vi "PAQ-Defragment.vi"() -> ()   [LabVIEW 2020, in "Sgraph_lib_V1.lvlib"]
uses:
  Builds/Sgraph_lib_V1.lvlib
  Controls/BIN-PAQ-Defrag-Attributes.ctl
  DBAL/controls/BIN/BINdata.ctl
  DBAL/DBAL-BIN.lvclass
panel:
  in  "Save Defragmented Files":bool
  out "error out":errorcluster
  out "XY Graph":cluster{dbl[], "data":dbl[]}(graph)
  out "Segments":string
  out "File name":string
  out "Folder name":string
  out "Table type":string
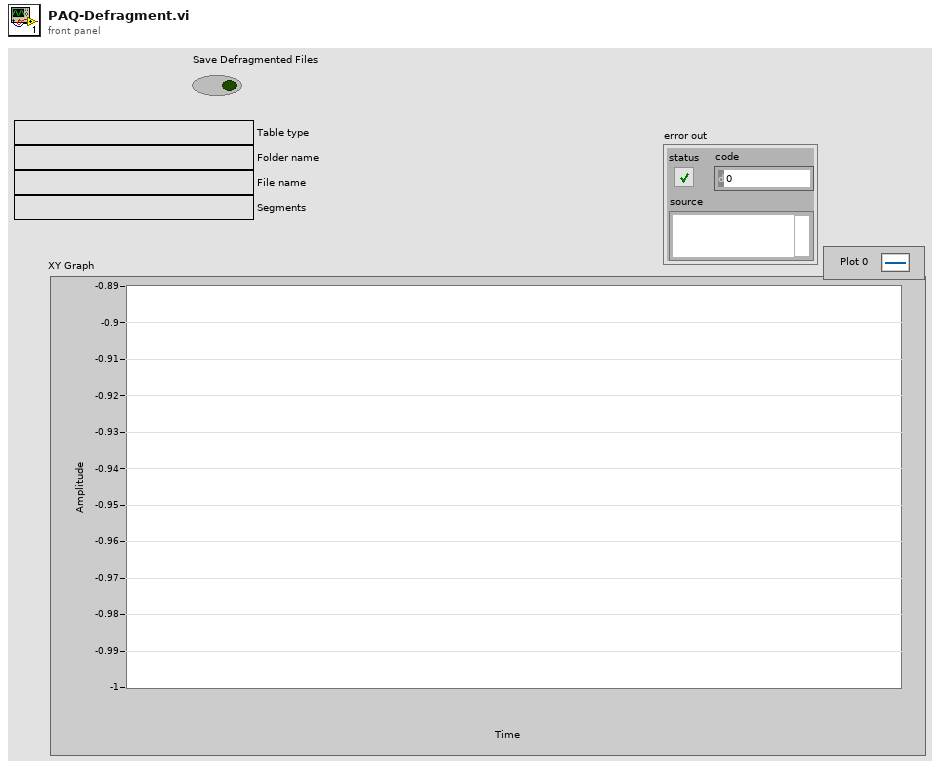
[diagram p1: front panel]
types:
  T1 = typedef "Sgraph_lib_V1.lvlib/BIN-PAQ-Defrag-Attributes.ctl" = cluster{"Database location":path, "Table Names":string[], "Ext":string, "WeekFolderNumbers":i32[], "FileDateNumbers":u64[], "WeekFolder":path, "HistFile":path, "BinHistData":T2, "Save Data":bool, "TAGs":string[], "Segments":i32}
  T2 = typedef "Sgraph_lib_V1.lvlib/DBAL-BIN.lvclass/BINdata.ctl" = cluster{"time":dbl[], "TagsData":cluster{"data":dbl[], "max":dbl[], "min":dbl[], "status":u32[]}[]}
  T3 = cluster{"data":dbl[], "max":dbl[], "min":dbl[], "status":u32[]}[]
  T4 = cluster{"data":dbl[], "max":dbl[], "min":dbl[], "status":u32[]}
  T5 = cluster{"TableName":string, "Data2save":cluster{"TAGs":string[], "time":dbl[], "TagsData":cluster{"data":dbl[], "max":dbl[], "min":dbl[], "status":u32[]}[]}}
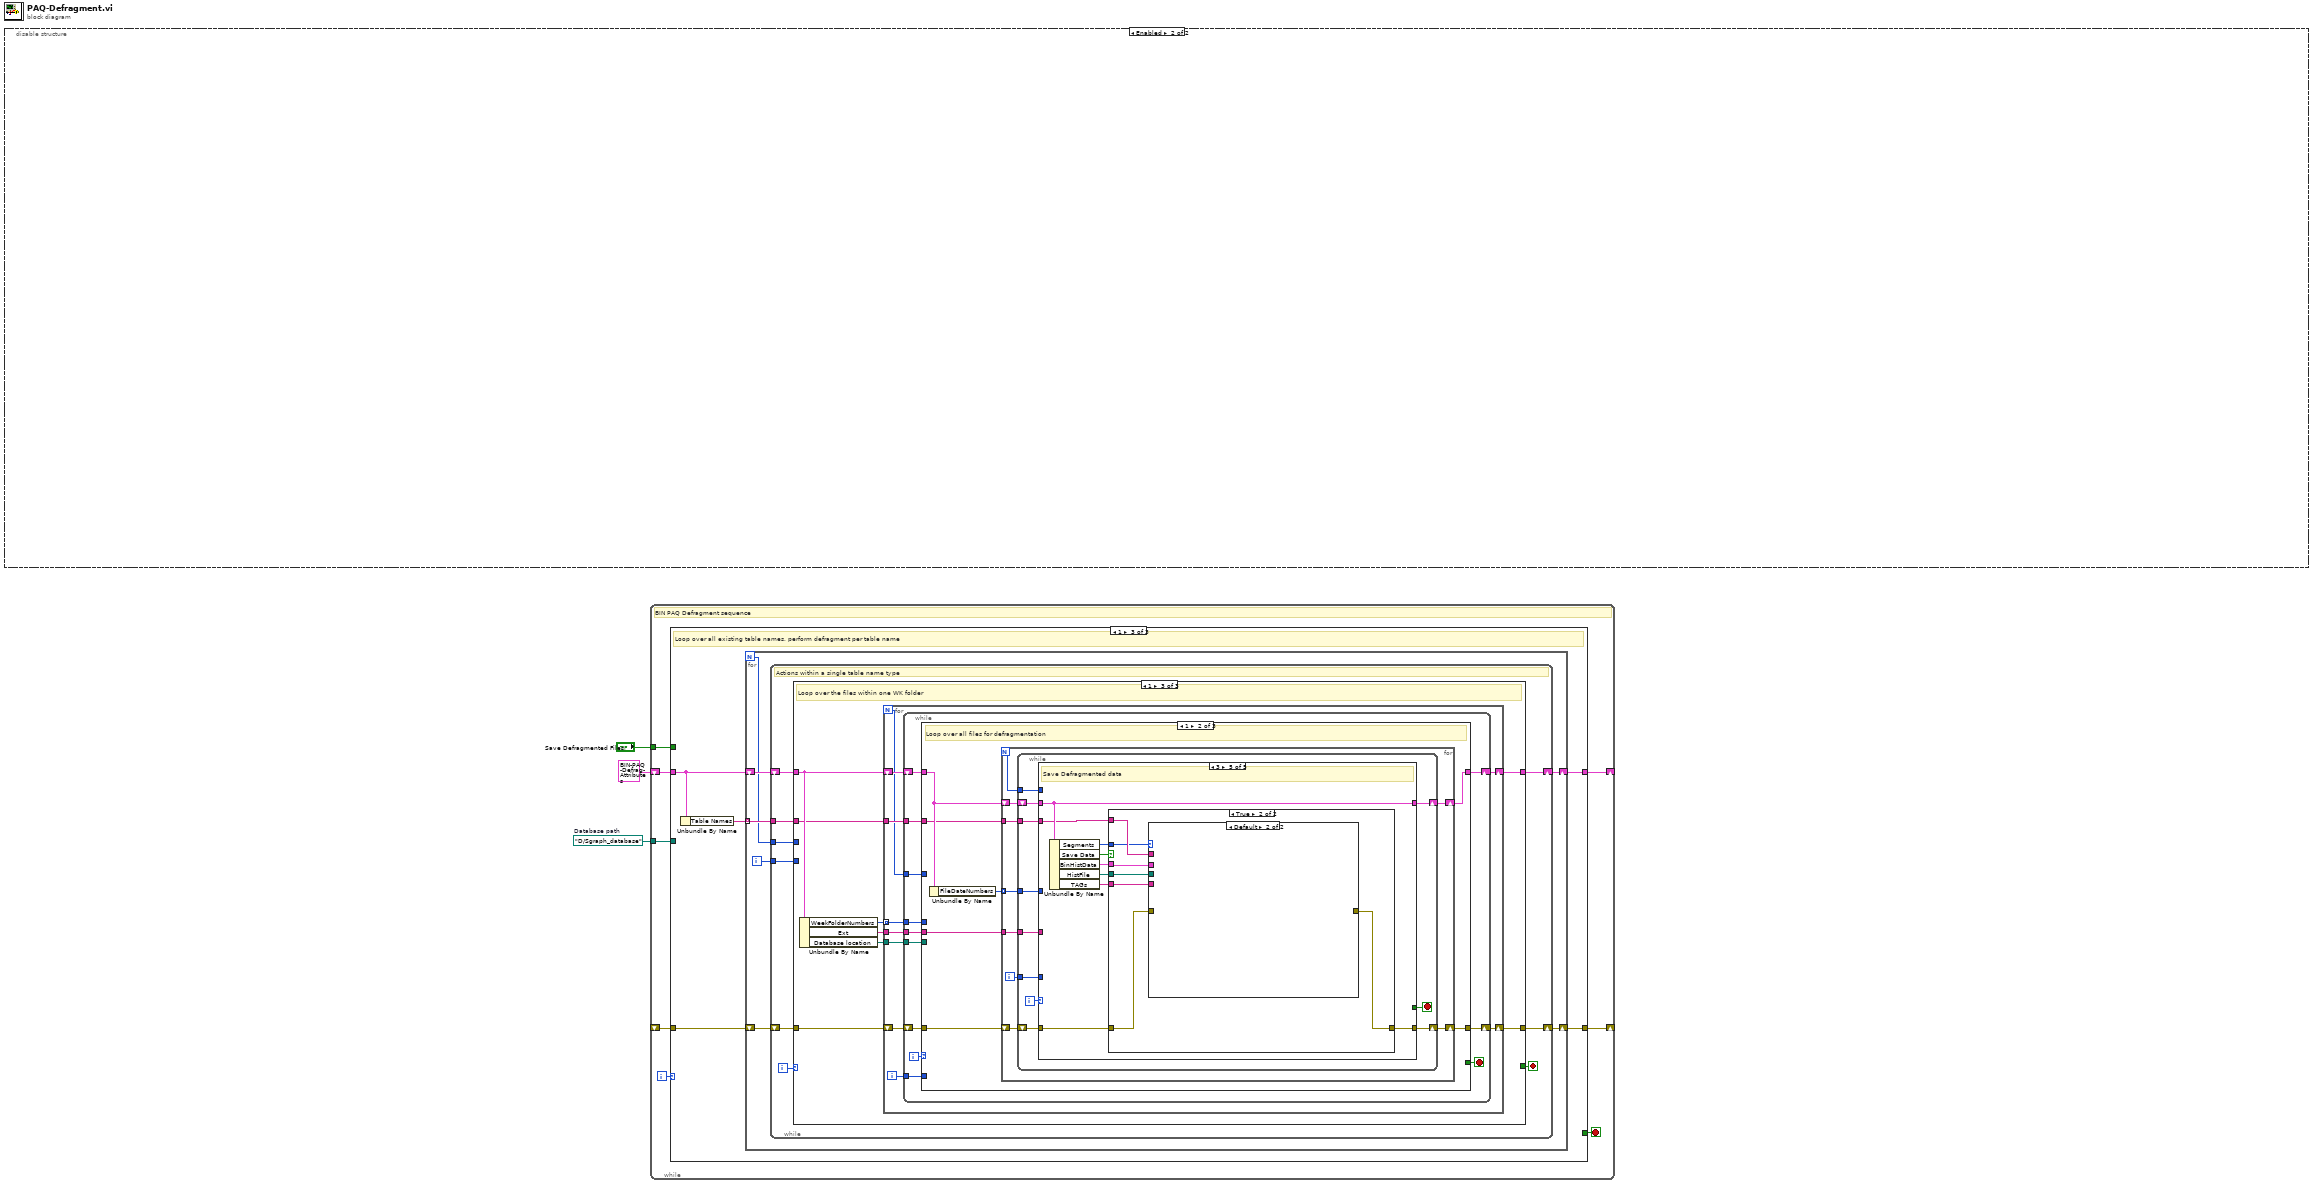
[diagram p0: block diagram]
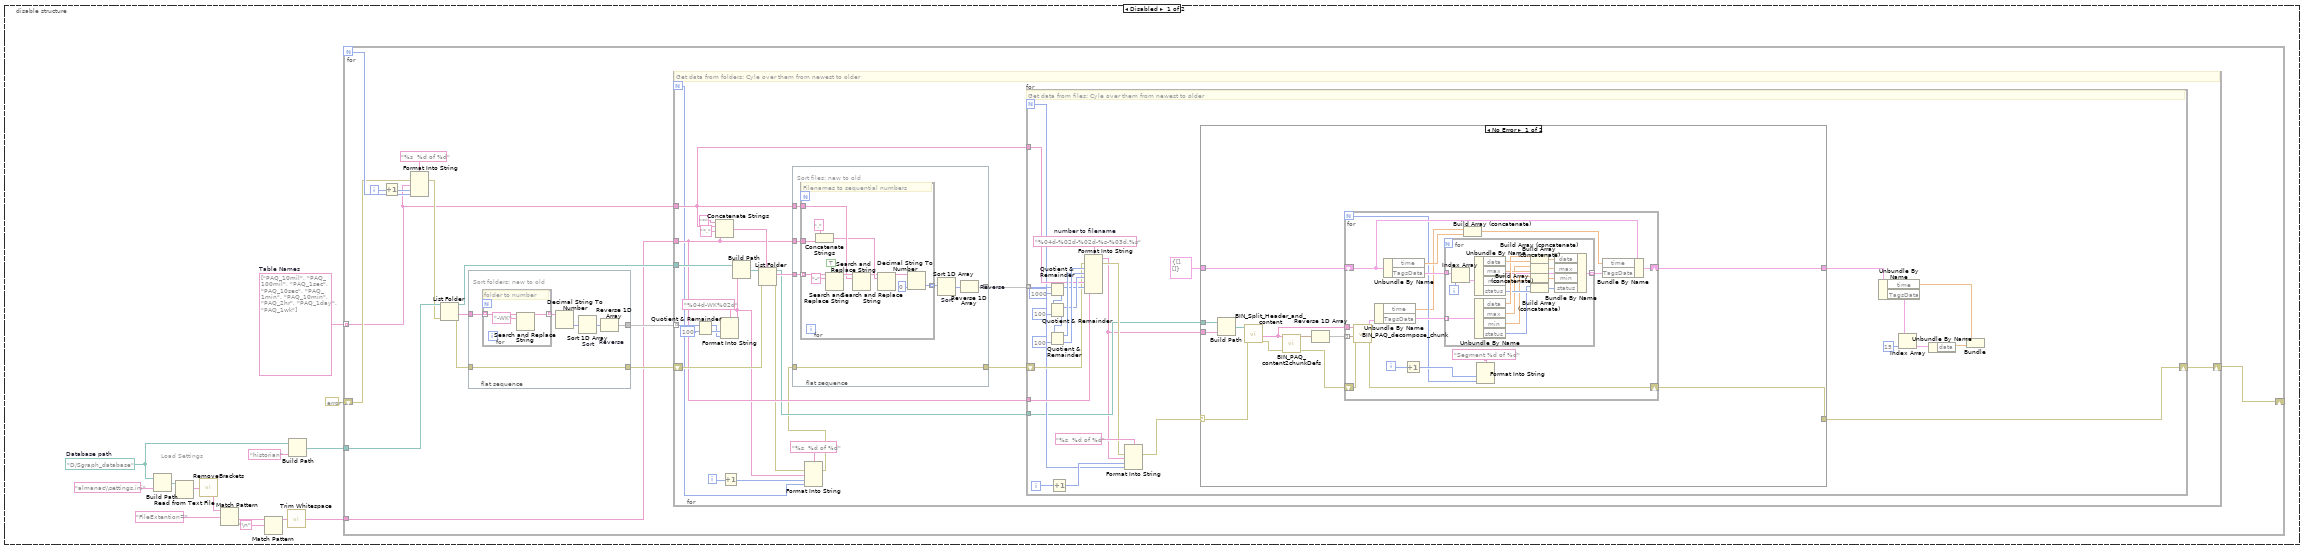
[diagram p2: hidden frame]
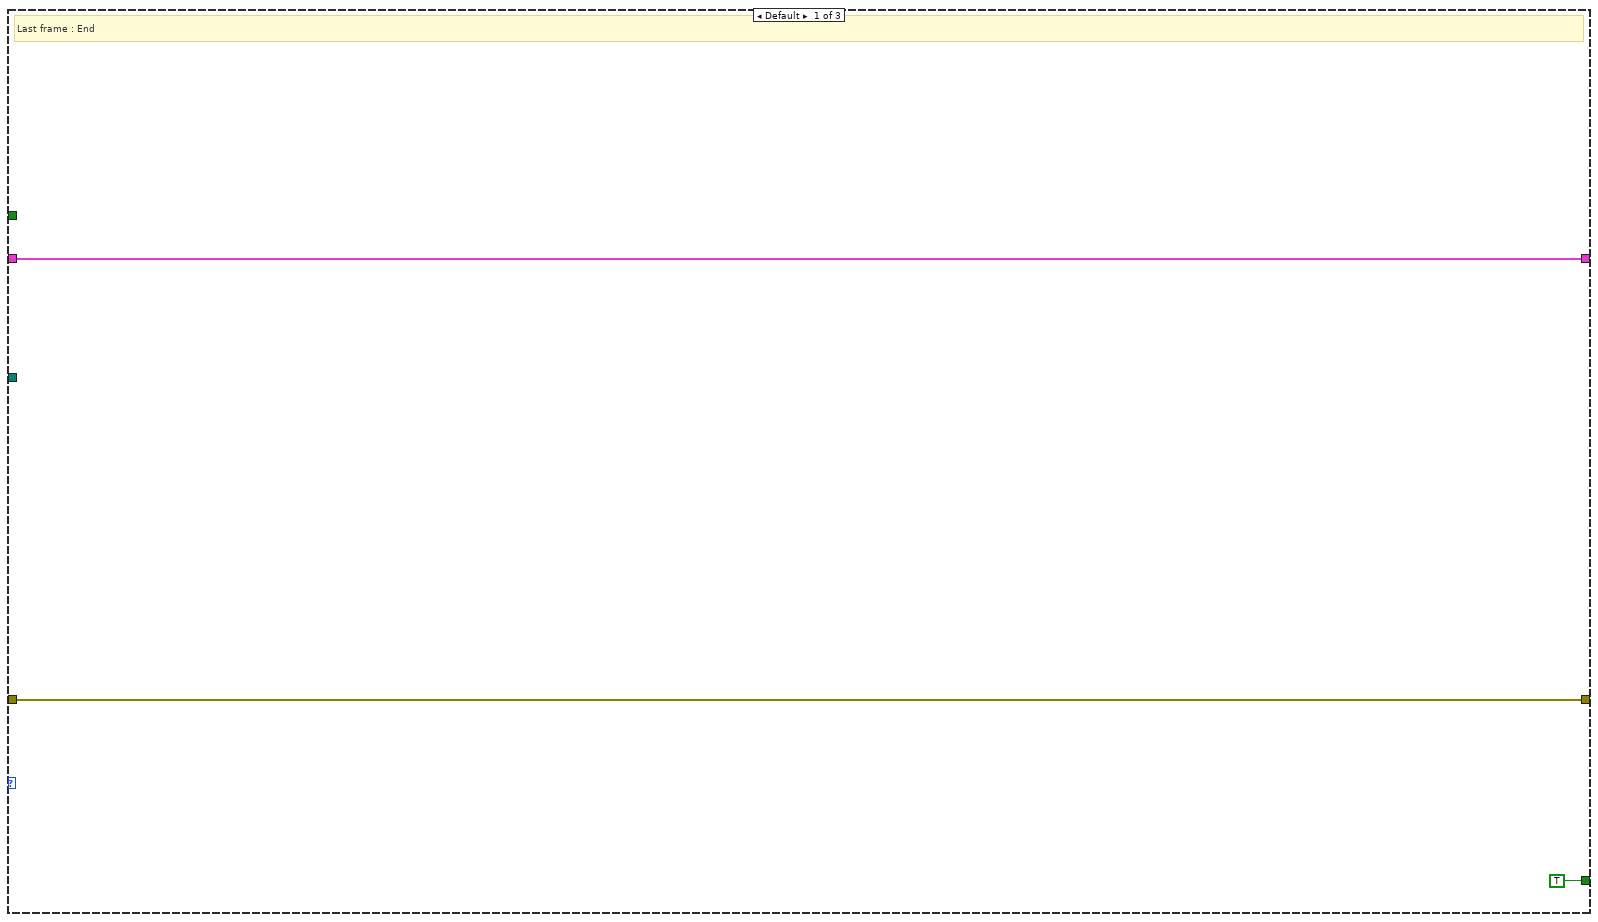
[diagram p4: hidden frame]
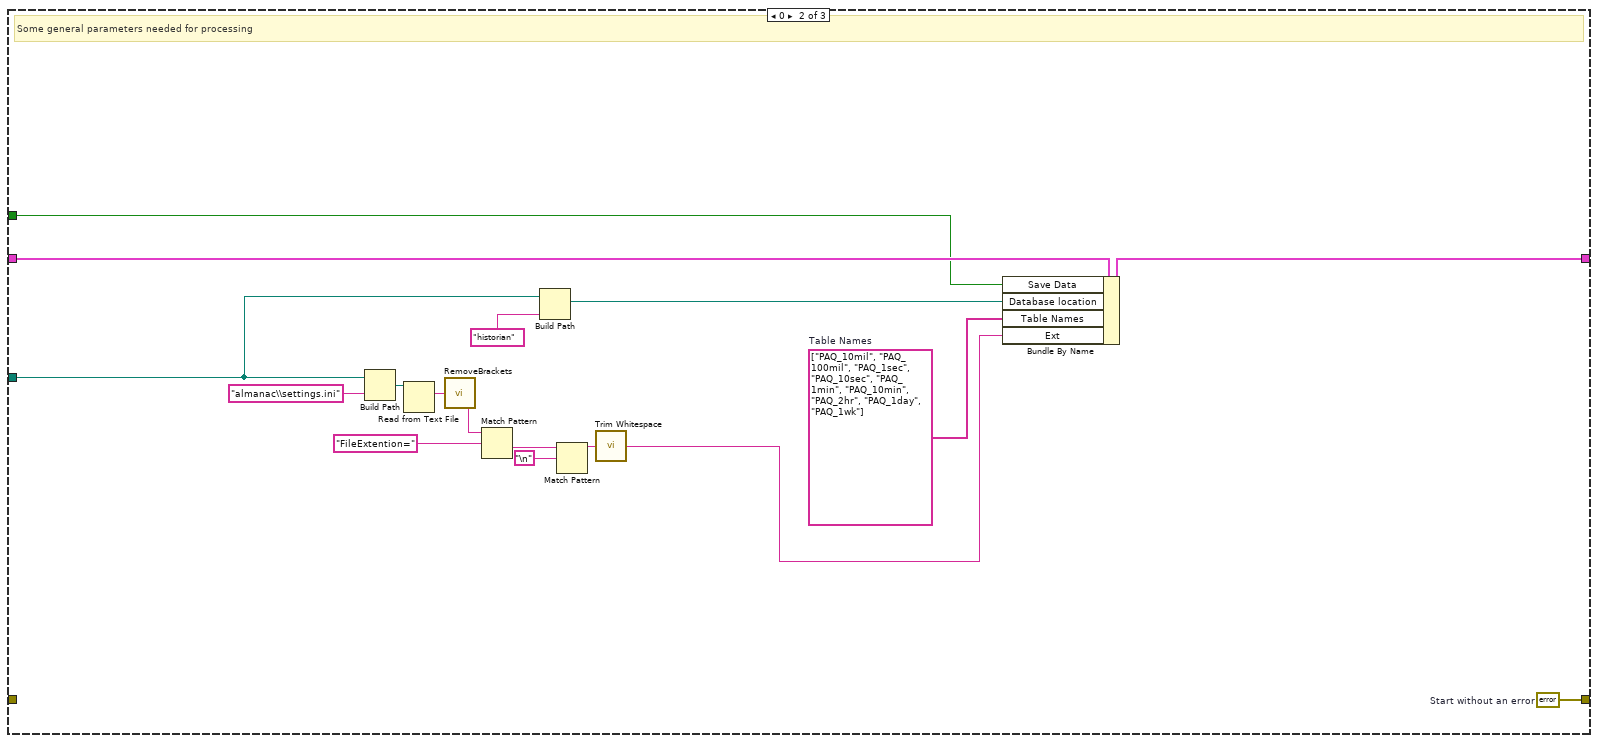
[diagram p5: hidden frame]
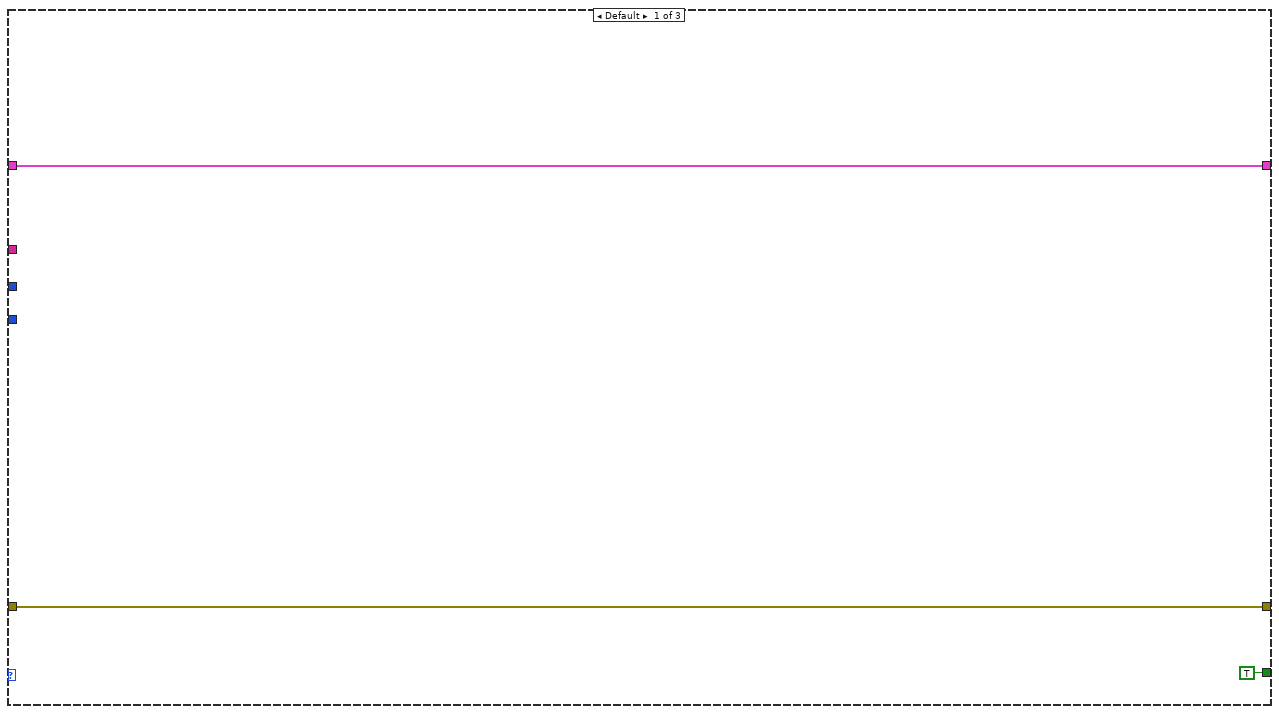
[diagram p6: hidden frame]
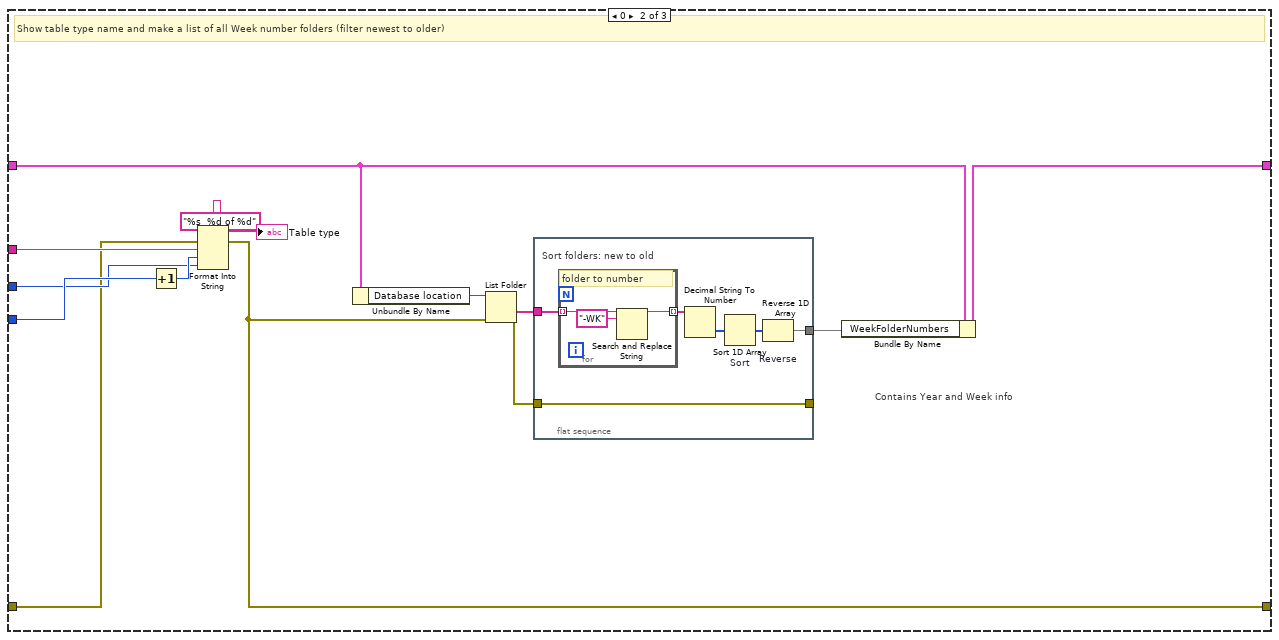
[diagram p7: hidden frame]
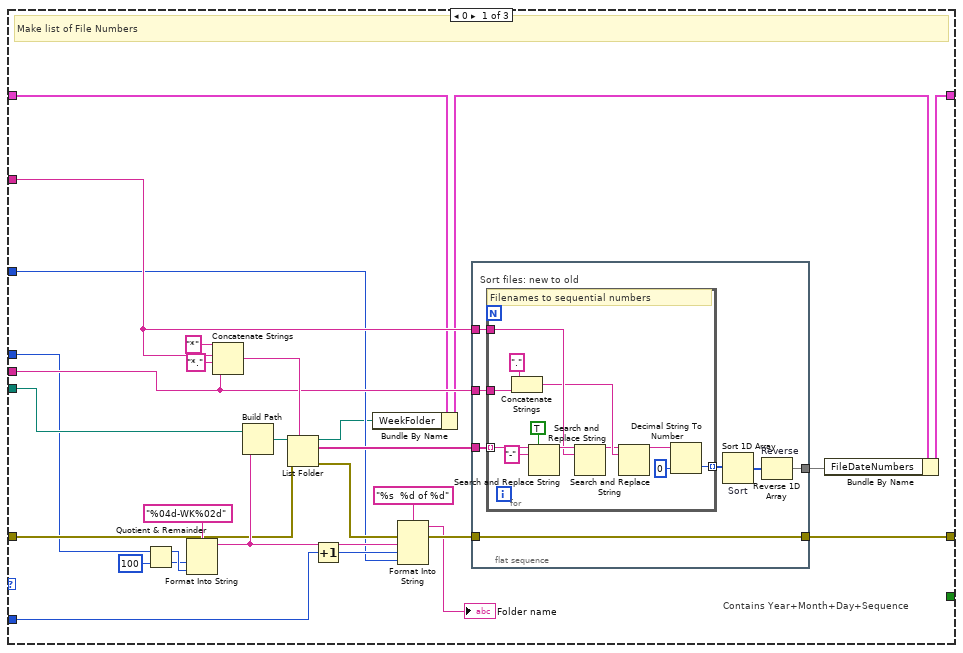
[diagram p8: hidden frame]
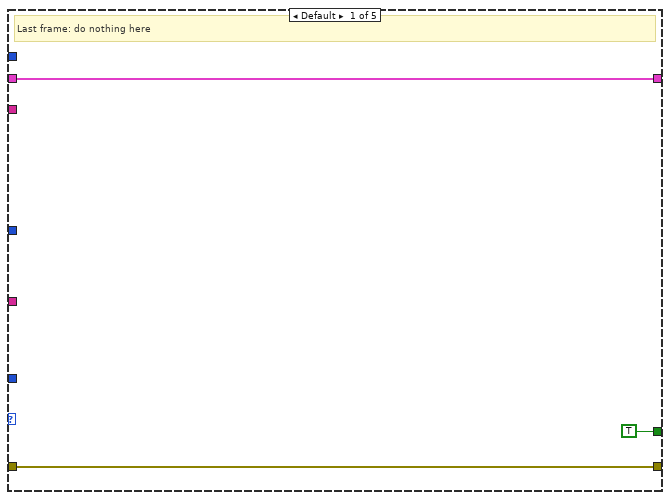
[diagram p9: hidden frame]
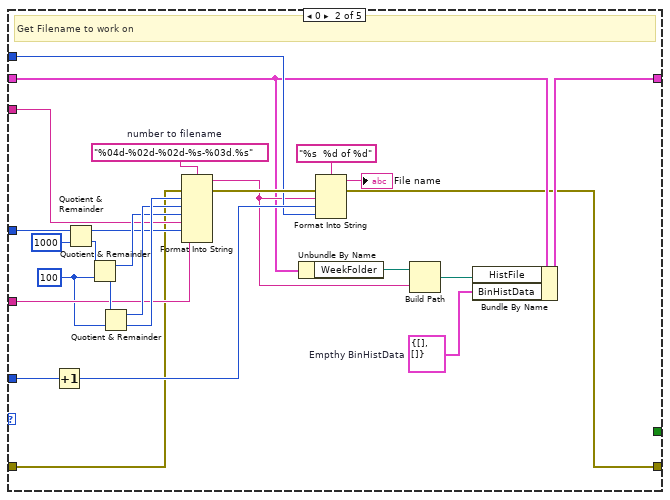
[diagram p10: hidden frame]
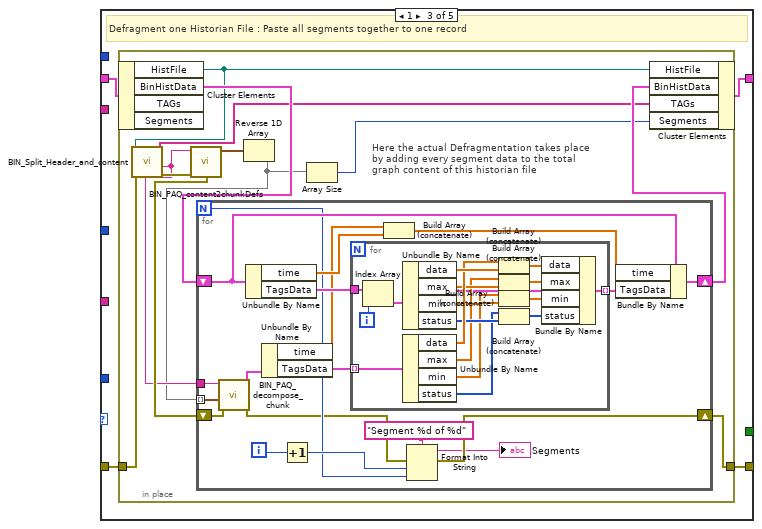
[diagram p11: hidden frame]
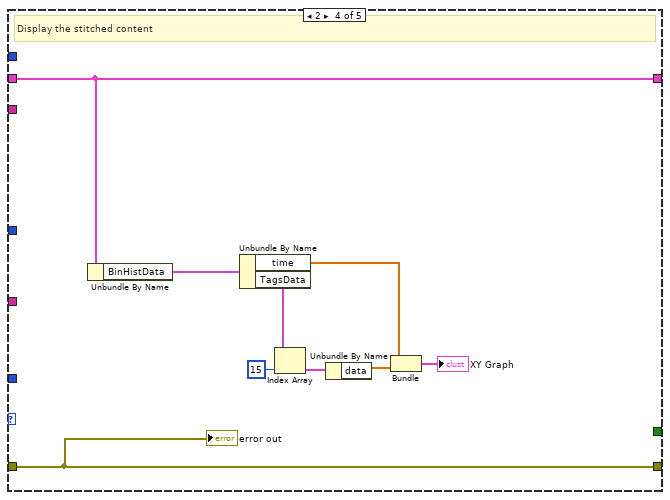
[diagram p12: hidden frame]
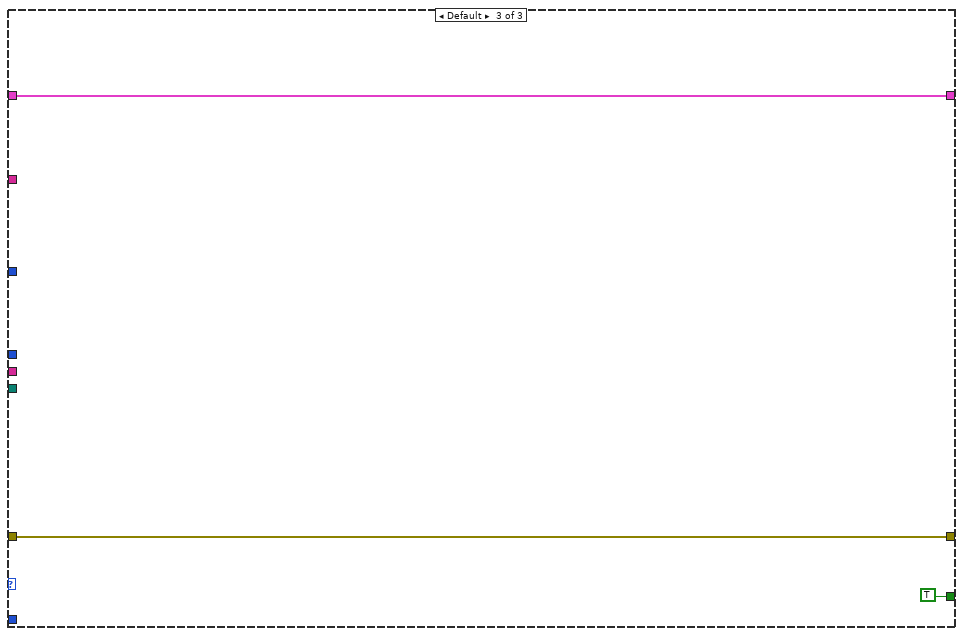
[diagram p15: hidden frame]
diagram:
  w3 = path "D:/Sgraph_database"  # Database path
  n1 = disable-structure shown="Enabled" {
    frame Disabled {
      w6 = path "D:/Sgraph_database"  # Database path
      w17 = string[] ["PAQ_10mil", "PAQ_100mil", "PAQ_1sec", "PAQ_10sec", "PAQ_1min", "PAQ_10min", "PAQ_2hr", "PAQ_1day", "PAQ_1wk"]  # Table Names
      # "Load Settings"
      n2 = Build Path(base path=w6, name or relative path="almanac\\settings.ini") -> (appended path=w14:path)
      n3 = Read from Text File(file (use dialog)=w14) -> (text=w15:string)  [unwired: 3 in, 3 out]
      n4 = call "RemoveBrackets.vi"("String in"=w15) -> ("String out"=w8:string)  [unwired: 6 in]
      n5 = Match Pattern(string=w8, regular expression="FileExtention=" ("format string")) -> (after substring=w12:string)  [unwired: 1 in, 3 out]
      n6 = Match Pattern(string=w12, regular expression="\n") -> (before substring=w9:string)  [unwired: 1 in, 3 out]
      n7 = call <vilib>:"Trim Whitespace.vi"("string"=w9) -> ("trimmed string"=w7:string)  [unwired: 1 in]
      n8 = Build Path(base path=w6, name or relative path="historian") -> (appended path=w4:path)
      n9 = for {
        N -> [w29]
        tunnel: w17 -> [w18] mode=indexing
        shift-right: [w22] -> _
        shift-left: errorcluster {"status"=FALSE, "code"=0, "source"=""} ("error IO") -> [w28]
        tunnel: w7 -> [w19]
        tunnel: w4 -> [w25]
        i -> [w31]
        n10 = Increment(x=w31) -> (x+1=w30:i32)
        n11 = Format Into String(format string="%s  %d of %d", error in=w28, w18, w30, w29) -> (error out=w24:errorcluster)  [unwired: 1 in, 1 out]
        n12 = List Folder(path=w25, error in=w24) -> (path out=w20:path, folder names=w26:string[], error out=w27:errorcluster)  [unwired: 2 in, 1 out]
        n13 = flat-sequence {
          tunnel: w26 -> [w159]
          tunnel: [w154] -> w21
          tunnel: w27 -> [w156]
          tunnel: [w156] -> w23
          frame #0 {
            # "Sort folders: new to old"
            n14 = for {
              tunnel: w159 -> [w162] mode=indexing
              tunnel: [w160] -> w158 mode=indexing
              # "folder to number"
              n15 = Search and Replace String(input string=w162, search string="-WK") -> (result string=w160:string)  [unwired: 6 in, 3 out]
            }
            n16 = Decimal String To Number ("to num")(string=w158) -> (number=w157:i32[])  [unwired: 2 in, 1 out]
            n17 = Sort 1D Array "Sort"(array=w157) -> (sorted array=w155:i32[])
            n18 = Reverse 1D Array "Reverse"(array=w155) -> (reversed array=w154:i32[])
          }
        }
        n19 = for {
          N -> [w35]
          shift-right: [w40] -> w22
          shift-left: w23 -> [w47]
          tunnel: w21 -> [w57] mode=indexing
          tunnel: w19 -> [w43]
          tunnel: w20 -> [w52]
          tunnel: w18 -> [w44]
          i -> [w37]
          # "Get data from folders: Cyle over them from newest to older"
          n20 = Quotient & Remainder(x=w57, y=100) -> (x-y*floor(x/y)=w53:i32, floor(x/y)=w54:i32)
          n21 = Concatenate Strings("*", w44, "*.", w43) -> (w48:string)
          n22 = Format Into String(format string="%04d-WK%02d", w54, w53) -> (resulting string=w38:string)  [unwired: 2 in, 1 out]
          n23 = Increment(x=w37) -> (x+1=w36:i32)
          n24 = Build Path(base path=w52, name or relative path=w38) -> (appended path=w51:path)
          n25 = List Folder(path=w51, pattern=w48, error in=w47) -> (path out=w42:path, filenames=w45:string[], error out=w34:errorcluster)  [unwired: 1 in, 1 out]
          n26 = flat-sequence {
            tunnel: w45 -> [w141]
            tunnel: w44 -> [w140]
            tunnel: w43 -> [w139]
            tunnel: [w136] -> w46
            tunnel: w33 -> [w135]
            tunnel: [w135] -> w41
            frame #0 {
              # "Sort files: new to old"
              n27 = for {
                tunnel: w141 -> [w142] mode=indexing
                tunnel: w140 -> [w150]
                tunnel: w139 -> [w149]
                tunnel: [w144] -> w137 mode=indexing
                # "Filenames to sequential numbers"
                n28 = Concatenate Strings("." ("string"), w149) -> (w148:string)
                n29 = Search and Replace String(replace all?=TRUE ("replace all? (F)"), input string=w142, search string="-") -> (result string=w151:string)  [unwired: 5 in, 3 out]
                n30 = Search and Replace String(input string=w151, search string=w150) -> (result string=w147:string)  [unwired: 6 in, 3 out]
                n31 = Search and Replace String(input string=w147, search string=w148) -> (result string=w145:string)  [unwired: 6 in, 3 out]
                n32 = Decimal String To Number(string=w145, default (0L)=u64 0 ("default (0 I32)")) -> (number=w144:u64)  [unwired: 1 in, 1 out]
              }
              n33 = Sort 1D Array "Sort"(array=w137) -> (sorted array=w138:u64[])
              n34 = Reverse 1D Array "Reverse"(array=w138) -> (reversed array=w136:u64[])
            }
          }
          n35 = Format Into String(format string="%s  %d of %d", error in=w34, w38, w36, w35) -> (error out=w33:errorcluster)  [unwired: 1 in, 1 out]
          n36 = for {
            N -> [w70]
            tunnel: w46 -> [w86] mode=indexing
            tunnel: w44 -> [w77]
            tunnel: w43 -> [w75]
            tunnel: w42 -> [w67]
            shift-right: [w65] -> w40
            shift-left: w41 -> [w74]
            i -> [w72]
            w81 = "%04d-%02d-%02d-%s-%03d.%s"  # number to filename
            # "Get data from files: Cyle over them from newest to older"
            n37 = Quotient & Remainder(x=w86, y=u64 1000) -> (x-y*floor(x/y)=w76:u64, floor(x/y)=w84:u64)
            n38 = Quotient & Remainder(x=w84, y=u64 100) -> (x-y*floor(x/y)=w78:u64, floor(x/y)=w82:u64)
            n39 = Quotient & Remainder(x=w82, y=u64 100) -> (x-y*floor(x/y)=w79:u64, floor(x/y)=w80:u64)
            n40 = Increment(x=w72) -> (x+1=w71:i32)
            n41 = Format Into String(format string=w81, error in=w74, w80, w79, w78, w77, w76, w75) -> (resulting string=w66:string, error out=w69:errorcluster)  [unwired: 1 in]
            n42 = Format Into String(format string="%s  %d of %d", error in=w69, w66, w71, w70) -> (error out=w68:errorcluster)  [unwired: 1 in, 1 out]
            n43 = case shown="No Error" w68 {
              selector: w68 -> [w98 w134]
              tunnel: [w94 w134] -> w65
              tunnel: w67 -> [w90 _]
              tunnel: w66 -> [w89 _]
              tunnel: [w91 _] -> w58
              tunnel: T2 {"time"=[], "TagsData"=[]} ("BinHistData") -> [w88 _]
              frame No Error {
                n44 = Build Path(base path=w90, name or relative path=w89) -> (appended path=w99:path)
                n45 = call "BIN_Split_Header_and_content.vi"("error in"=w98, "Path in"=w99) -> ("error out"=w97:errorcluster, "Content"=w96:string)  [unwired: 5 in, 3 out]
                n46 = call "BIN_PAQ_content2chunkDefs.vi"("error in (no error)"=w97, "Content"=w96) -> ("error out"=w95:errorcluster, "Data segments"=w93:cluster{"Offset":u32, "Size":u32}[])  [unwired: 8 in]
                n47 = Reverse 1D Array(array=w93) -> (reversed array=w92:cluster{"Offset":u32, "Size":u32}[])
                n48 = for {
                  N -> [w101]
                  tunnel: w92 -> [w116] mode=indexing
                  tunnel: w96 -> [w115]
                  shift-right: [w113] -> w94
                  shift-left: w95 -> [w114]
                  shift-right: [w110] -> w91
                  shift-left: w88 -> [w112]
                  i -> [w103]
                  n49 = call "BIN_PAQ_decompose_chunk.vi"("error in (no error)"=w114, "Offset"=w116, "Content"=w115) -> ("error out"=w113:errorcluster, "PAQ_data"=w111:T2)  [unwired: 6 in, 1 out]
                  n50 = Unbundle By Name(w111) -> ("time"=w100:dbl[], "TagsData"=w108:T3)
                  n51 = Unbundle By Name(w112) -> ("time"=w109:dbl[], "TagsData"=w107:T3)
                  n52 = Increment(x=w103) -> (x+1=w102:i32)
                  n53 = for {
                    tunnel: w108 -> [w131] mode=indexing
                    tunnel: w107 -> [w133]
                    tunnel: [w121] -> w106 mode=indexing
                    i -> [w132]
                    n54 = Index Array(array=w133, index=w132) -> (element=w122:T4)
                    n55 = Unbundle By Name(w122) -> ("data"=w130:dbl[], "max"=w128:dbl[], "min"=w127:dbl[], "status"=w126:u32[])
                    n56 = Unbundle By Name(w131) -> ("data"=w129:dbl[], "max"=w123:dbl[], "min"=w124:dbl[], "status"=w125:u32[])
                    n57 = Build Array (concatenate)(w129, w130) -> (w118:dbl[])
                    n58 = Build Array (concatenate)(w123, w128) -> (w119:dbl[])
                    n59 = Build Array (concatenate)(w124, w127) -> (w120:dbl[])
                    n60 = Build Array (concatenate)(w125, w126) -> (w117:u32[])
                    n61 = Bundle By Name(cluster=w122, "data"=w118, "max"=w119, "min"=w120, "status"=w117) -> (w121:T4)
                  }
                  n62 = Build Array (concatenate)(w100, w109) -> (w105:dbl[])
                  n63 = Format Into String(format string="Segment %d of %d", w102, w101) -> ()  [unwired: 2 in, 2 out]
                  n64 = Bundle By Name(cluster=w112, "time"=w105, "TagsData"=w106) -> (w110:T2)
                }
              }
              frame Error {
              }
            }
            n65 = Unbundle By Name(w58) -> ("time"=w61:dbl[], "TagsData"=w60:T3)
            n66 = Index Array(array=w60, index=15) -> (element=w62:T4)
            n67 = Unbundle By Name(w62) -> ("data"=w63:dbl[])
            n68 = Bundle("time"=w61, "data"=w63) -> ()  [unwired: 1 in, 1 out]
          }
        }
      }
    }
    frame Enabled {
    }
  }
  n69 = while {
    tunnel: w3 -> [w168]
    shift-right: [w166] -> _
    shift-left: T1 {"Database location"=path "", "Table Names"=["PAQ_10mil", "PAQ_100mil", "PAQ_1sec", "PAQ_10sec", "PAQ_1min", "PAQ_10min", "PAQ_2hr", "PAQ_1day", "PAQ_1wk"], "Ext"="", "WeekFolderNumbers"=[], "FileDateNumbers"=[], "WeekFolder"=path "", "HistFile"=path "", "BinHistData"={"time"=[], "TagsData"=[]}, "Save Data"=FALSE, "TAGs"=[], "Segments"=0} ("Defrag-attr") -> [w167]
    shift-right: [w165] -> _
    shift-left: _ -> [w164]
    tunnel: "Save Defragmented Files" -> [w163]
    i -> [w170]
    stop <- w169 stop-if-true
    # "BIN PAQ Defragment sequence"
    n70 = case shown="1" w170 {
      tunnel: [TRUE _ _] -> w169
      tunnel: w168 -> [_ w179 _]
      tunnel: w167 -> [w173 w182 w194]
      tunnel: [w173 w181 w195] -> w166
      tunnel: [w172 w175 w191] -> w165
      tunnel: w164 -> [w172 _ w192]
      tunnel: w163 -> [_ w174 _]
      frame Default {
        # "Last frame : End"
      }
      frame 0 {
        w175 = errorcluster {"status"=FALSE, "code"=0, "source"=""}  # Start without an error
        w177 = string[] ["PAQ_10mil", "PAQ_100mil", "PAQ_1sec", "PAQ_10sec", "PAQ_1min", "PAQ_10min", "PAQ_2hr", "PAQ_1day", "PAQ_1wk"]  # Table Names
        # "Some general parameters needed for processing"
        n71 = Build Path(base path=w179, name or relative path="almanac\\settings.ini") -> (appended path=w184:path)
        n72 = Read from Text File(file (use dialog)=w184) -> (text=w183:string)  [unwired: 3 in, 3 out]
        n73 = call "RemoveBrackets.vi"("String in"=w183) -> ("String out"=w190:string)  [unwired: 6 in]
        n74 = Match Pattern(string=w190, regular expression="FileExtention=" ("format string")) -> (after substring=w186:string)  [unwired: 1 in, 3 out]
        n75 = Build Path(base path=w179, name or relative path="historian") -> (appended path=w178:path)
        n76 = Match Pattern(string=w186, regular expression="\n") -> (before substring=w189:string)  [unwired: 1 in, 3 out]
        n77 = call <vilib>:"Trim Whitespace.vi"("string"=w189) -> ("trimmed string"=w176:string)  [unwired: 1 in]
        n78 = Bundle By Name(cluster=w182, "Save Data"=w174, "Database location"=w178, "Table Names"=w177, "Ext"=w176) -> (w181:T1)
      }
      frame 1 {
        # "Loop over all existing table names, perform defragment per table name"
        n79 = Unbundle By Name(w194) -> ("Table Names"=w193:string[])
        n80 = for {
          N -> [w198]
          shift-right: [w201] -> w195
          shift-left: w194 -> [w202]
          tunnel: w193 -> [w200] mode=indexing
          shift-right: [w196] -> w191
          shift-left: w192 -> [w197]
          i -> [w199]
          # "Loop over all existing table names, perform defragment per table name"
          n81 = while {
            shift-right: [w208] -> w201
            shift-left: w202 -> [w209]
            tunnel: w200 -> [w206]
            tunnel: w199 -> [w207]
            tunnel: w198 -> [w205]
            shift-right: [w203] -> w196
            shift-left: w197 -> [w204]
            i -> [w211]
            stop <- w210 stop-if-true
            # "Actions within a single table name type"
            n82 = case shown="1" w211 {
              tunnel: [TRUE _ _] -> w210
              tunnel: w209 -> [w213 w215 w245]
              tunnel: [w213 w216 w244] -> w208
              tunnel: w207 -> [_ w226 _]
              tunnel: w206 -> [_ w225 w241]
              tunnel: w205 -> [_ w224 _]
              tunnel: w204 -> [w212 w222 w243]
              tunnel: [w212 w219 w242] -> w203
              frame Default {
              }
              frame 0 {
                # "Contains Year and Week info"
                # "Show table type name and make a list of all Week number folders (filter newest to older)"
                n83 = Increment(x=w226) -> (x+1=w227:i32)
                n84 = Format Into String(format string="%s  %d of %d", error in=w222, w225, w227, w224) -> (resulting string=→"Table type":string, error out=w219:errorcluster)  [unwired: 1 in]
                n85 = Unbundle By Name(w215) -> ("Database location"=w218:path)
                n86 = List Folder(path=w218, error in=w219) -> (folder names=w221:string[], error out=w220:errorcluster)  [unwired: 2 in, 2 out]
                n87 = flat-sequence {
                  tunnel: w221 -> [w234]
                  tunnel: [w229] -> w217
                  tunnel: w220 -> [w231]
                  tunnel: [w231] -> _
                  frame #0 {
                    # "Sort folders: new to old"
                    n88 = for {
                      tunnel: w234 -> [w237] mode=indexing
                      tunnel: [w235] -> w233 mode=indexing
                      # "folder to number"
                      n89 = Search and Replace String(input string=w237, search string="-WK") -> (result string=w235:string)  [unwired: 6 in, 3 out]
                    }
                    n90 = Decimal String To Number ("to num")(string=w233) -> (number=w232:i32[])  [unwired: 2 in, 1 out]
                    n91 = Sort 1D Array "Sort"(array=w232) -> (sorted array=w230:i32[])
                    n92 = Reverse 1D Array "Reverse"(array=w230) -> (reversed array=w229:i32[])
                  }
                }
                n93 = Bundle By Name(cluster=w215, "WeekFolderNumbers"=w217) -> (w216:T1)
              }
              frame 1 {
                # "Loop over the files within one WK folder"
                n94 = Unbundle By Name(w245) -> ("WeekFolderNumbers"=w238:i32[], "Ext"=w240:string, "Database location"=w239:path)
                n95 = for {
                  N -> [w246]
                  tunnel: w238 -> [w248] mode=indexing
                  shift-right: [w253] -> w244
                  shift-left: w245 -> [w255]
                  shift-right: [w252] -> w242
                  shift-left: w243 -> [w254]
                  tunnel: w241 -> [w251]
                  tunnel: w240 -> [w250]
                  tunnel: w239 -> [w249]
                  i -> [w247]
                  n96 = while {
                    shift-right: [w264] -> w252
                    shift-left: w254 -> [w266]
                    shift-right: [w263] -> w253
                    shift-left: w255 -> [w267]
                    tunnel: w251 -> [w261]
                    tunnel: w250 -> [w260]
                    tunnel: w249 -> [w259]
                    tunnel: w248 -> [w258]
                    tunnel: w247 -> [w257]
                    tunnel: w246 -> [w256]
                    i -> [w265]
                    stop <- w262 stop-if-true
                    n97 = case shown="1" w265 {
                      tunnel: w267 -> [w268 w320 w463]
                      tunnel: w266 -> [w278 w318 w464]
                      tunnel: [w273 w317 w464] -> w264
                      tunnel: [w272 w319 w463] -> w263
                      tunnel: [_ _ TRUE] -> w262
                      tunnel: w261 -> [w281 w316 _]
                      tunnel: w260 -> [w280 w315 _]
                      tunnel: w259 -> [w279 _ _]
                      tunnel: w258 -> [w277 _ _]
                      tunnel: w257 -> [w276 _ _]
                      tunnel: w256 -> [w275 _ _]
                      frame 0 {
                        # "Contains Year+Month+Day+Sequence"
                        # "Make list of File Numbers"
                        n98 = Quotient & Remainder(x=w277, y=100) -> (x-y*floor(x/y)=w288:i32, floor(x/y)=w287:i32)
                        n99 = Format Into String(format string="%04d-WK%02d", w287, w288) -> (resulting string=w292:string)  [unwired: 2 in, 1 out]
                        n100 = Concatenate Strings("*", w281, "*.", w280) -> (w290:string)
                        n101 = Build Path(base path=w279, name or relative path=w292) -> (appended path=w289:path)
                        n102 = List Folder(path=w289, pattern=w290, error in=w278) -> (path out=w270:path, filenames=w291:string[], error out=w294:errorcluster)  [unwired: 1 in, 1 out]
                        n103 = Increment(x=w276) -> (x+1=w293:i32)
                        n104 = Bundle By Name(cluster=w268, "WeekFolder"=w270) -> (w269:T1)
                        n105 = Format Into String(format string="%s  %d of %d", error in=w294, w292, w293, w275) -> (resulting string=→"Folder name":string, error out=w295:errorcluster)  [unwired: 1 in]
                        n106 = flat-sequence {
                          tunnel: w291 -> [w302]
                          tunnel: w281 -> [w301]
                          tunnel: w280 -> [w300]
                          tunnel: [w297] -> w271
                          tunnel: w295 -> [w296]
                          tunnel: [w296] -> w273
                          frame #0 {
                            # "Sort files: new to old"
                            n107 = for {
                              tunnel: w302 -> [w303] mode=indexing
                              tunnel: w301 -> [w311]
                              tunnel: w300 -> [w310]
                              tunnel: [w305] -> w298 mode=indexing
                              # "Filenames to sequential numbers"
                              n108 = Concatenate Strings("." ("string"), w310) -> (w309:string)
                              n109 = Search and Replace String(replace all?=TRUE ("replace all? (F)"), input string=w303, search string="-") -> (result string=w312:string)  [unwired: 5 in, 3 out]
                              n110 = Search and Replace String(input string=w312, search string=w311) -> (result string=w308:string)  [unwired: 6 in, 3 out]
                              n111 = Search and Replace String(input string=w308, search string=w309) -> (result string=w306:string)  [unwired: 6 in, 3 out]
                              n112 = Decimal String To Number(string=w306, default (0L)=u64 0 ("default (0 I32)")) -> (number=w305:u64)  [unwired: 1 in, 1 out]
                            }
                            n113 = Sort 1D Array "Sort"(array=w298) -> (sorted array=w299:u64[])
                            n114 = Reverse 1D Array "Reverse"(array=w299) -> (reversed array=w297:u64[])
                          }
                        }
                        n115 = Bundle By Name(cluster=w269, "FileDateNumbers"=w271) -> (w272:T1)
                      }
                      frame 1 {
                        # "Loop over all files for defragmentation"
                        n116 = Unbundle By Name(w320) -> ("FileDateNumbers"=w321:u64[])
                        n117 = for {
                          N -> [w323]
                          tunnel: w321 -> [w326] mode=indexing
                          shift-right: [w322] -> w319
                          shift-left: w320 -> [w330]
                          shift-right: [w328] -> w317
                          shift-left: w318 -> [w329]
                          tunnel: w316 -> [w327]
                          tunnel: w315 -> [w325]
                          i -> [w324]
                          n118 = while {
                            shift-right: [w337] -> w322
                            shift-left: w330 -> [w340]
                            shift-right: [w338] -> w328
                            shift-left: w329 -> [w339]
                            tunnel: w327 -> [w335]
                            tunnel: w326 -> [w334]
                            tunnel: w325 -> [w333]
                            tunnel: w324 -> [w332]
                            tunnel: w323 -> [w331]
                            i -> [w341]
                            stop <- w336 stop-if-true
                            n119 = case shown="3" w341 {
                              tunnel: w340 -> [w342 w348 w374 w424 w440]
                              tunnel: w339 -> [w344 w346 w373 w423 w438]
                              tunnel: [w344 w347 w372 w423 w437] -> w338
                              tunnel: [w342 w349 w371 w424 w440] -> w337
                              tunnel: [TRUE _ _ _ _] -> w336
                              tunnel: w335 -> [_ w360 _ _ w433]
                              tunnel: w334 -> [_ w359 _ _ _]
                              tunnel: w333 -> [_ w358 _ _ _]
                              tunnel: w332 -> [_ w356 _ _ _]
                              tunnel: w331 -> [_ w354 _ _ _]
                              frame Default {
                                # "Last frame: do nothing here"
                              }
                              frame 0 {
                                w345 = T2 {"time"=[], "TagsData"=[]}  # Empthy BinHistData
                                w362 = "%04d-%02d-%02d-%s-%03d.%s"  # number to filename
                                w357 = u64 100 ("y")
                                # "Get Filename to work on"
                                n120 = Increment(x=w356) -> (x+1=w355:i32)
                                n121 = Quotient & Remainder(x=w359, y=u64 1000) -> (x-y*floor(x/y)=w365:u64, floor(x/y)=w370:u64)
                                n122 = Quotient & Remainder(x=w370, y=w357) -> (x-y*floor(x/y)=w366:u64, floor(x/y)=w369:u64)
                                n123 = Quotient & Remainder(x=w369, y=w357) -> (x-y*floor(x/y)=w367:u64, floor(x/y)=w368:u64)
                                n124 = Format Into String(format string=w362, error in=w346, w368, w367, w366, w360, w365, w358) -> (resulting string=w351:string, error out=w364:errorcluster)  [unwired: 1 in]
                                n125 = Unbundle By Name(w348) -> ("WeekFolder"=w352:path)
                                n126 = Format Into String(format string="%s  %d of %d", error in=w364, w351, w355, w354) -> (resulting string=→"File name":string, error out=w347:errorcluster)  [unwired: 1 in]
                                n127 = Build Path(base path=w352, name or relative path=w351) -> (appended path=w350:path)
                                n128 = Bundle By Name(cluster=w348, "HistFile"=w350, "BinHistData"=w345) -> (w349:T1)
                              }
                              frame 1 {
                                # "Defragment one Historian File : Paste all segments together to one record"
                                n129 = in-place {
                                in-place-border: w373 -> [w384]
                                in-place-border: [w379] -> w372
                                # "Here the actual Defragmentation takes place\nby adding every segment data to the total\ngraph content of this historian file"
                                n130 = in-place-cluster #1(w374) -> ("HistFile"=w378:path, "BinHistData"=w381:T2)  [unwired: 2 out]
                                n131 = call "BIN_Split_Header_and_content.vi"("error in"=w384, "Path in"=w378) -> ("error out"=w385:errorcluster, "Content"=w382:string, "TAGs"=w377:string[])  [unwired: 5 in, 2 out]
                                n132 = call "BIN_PAQ_content2chunkDefs.vi"("error in (no error)"=w385, "Content"=w382) -> ("error out"=w383:errorcluster, "Data segments"=w386:cluster{"Offset":u32, "Size":u32}[])  [unwired: 8 in]
                                n133 = Reverse 1D Array(array=w386) -> (reversed array=w376:cluster{"Offset":u32, "Size":u32}[])
                                n134 = for {
                                N -> [w391]
                                tunnel: w376 -> [w405] mode=indexing
                                tunnel: w382 -> [w404]
                                shift-right: [w388] -> w379
                                shift-left: w383 -> [w403]
                                shift-right: [w400] -> w380
                                shift-left: w381 -> [w402]
                                i -> [w393]
                                n135 = call "BIN_PAQ_decompose_chunk.vi"("error in (no error)"=w403, "Offset"=w405, "Content"=w404) -> ("error out"=w389:errorcluster, "PAQ_data"=w401:T2)  [unwired: 6 in, 1 out]
                                n136 = Unbundle By Name(w402) -> ("time"=w399:dbl[], "TagsData"=w397:T3)
                                n137 = Unbundle By Name(w401) -> ("time"=w390:dbl[], "TagsData"=w398:T3)
                                n138 = Increment(x=w393) -> (x+1=w392:i32)
                                n139 = for {
                                tunnel: w398 -> [w420] mode=indexing
                                tunnel: w397 -> [w422]
                                tunnel: [w410] -> w396 mode=indexing
                                i -> [w421]
                                n140 = Index Array(array=w422, index=w421) -> (element=w411:T4)
                                n141 = Unbundle By Name(w411) -> ("data"=w419:dbl[], "max"=w417:dbl[], "min"=w416:dbl[], "status"=w415:u32[])
                                n142 = Unbundle By Name(w420) -> ("data"=w418:dbl[], "max"=w412:dbl[], "min"=w413:dbl[], "status"=w414:u32[])
                                n143 = Build Array (concatenate)(w418, w419) -> (w407:dbl[])
                                n144 = Build Array (concatenate)(w412, w417) -> (w408:dbl[])
                                n145 = Build Array (concatenate)(w413, w416) -> (w409:dbl[])
                                n146 = Build Array (concatenate)(w414, w415) -> (w406:u32[])
                                n147 = Bundle By Name(cluster=w411, "data"=w407, "max"=w408, "min"=w409, "status"=w406) -> (w410:T4)
                                }
                                n148 = Build Array (concatenate)(w390, w399) -> (w395:dbl[])
                                n149 = Format Into String(format string="Segment %d of %d", error in=w389, w392, w391) -> (resulting string=→"Segments":string, error out=w388:errorcluster)  [unwired: 1 in]
                                n150 = Bundle By Name(cluster=w402, "time"=w395, "TagsData"=w396) -> (w400:T2)
                                }
                                n151 = Array Size(array=w376) -> (size(s)=w375:i32)
                                n152 = in-place-cluster #1("HistFile"=w378, "BinHistData"=w380, "TAGs"=w377, "Segments"=w375) -> (w371:T1)
                                }
                              }
                              frame 2 {
                                # "Display the stitched content"
                                n153 = Unbundle By Name(w424) -> ("BinHistData"=w426:T2)
                                n154 = Unbundle By Name(w426) -> ("time"=w429:dbl[], "TagsData"=w428:T3)
                                n155 = Index Array(array=w428, index=15) -> (element=w430:T4)
                                n156 = Unbundle By Name(w430) -> ("data"=w431:dbl[])
                                n157 = Bundle("time"=w429, "data"=w431) -> (→"XY Graph":cluster{"time":dbl[], "data":dbl[]})  [unwired: 1 in]
                                "error out" <- w423
                              }
                              frame 3 {
                                # "Save Defragmented data"
                                n158 = Unbundle By Name(w440) -> ("Segments"=w432:i32, "Save Data"=w439:bool, "BinHistData"=w436:T2, "HistFile"=w435:path, "TAGs"=w434:string[])
                                n159 = case shown="True" w439 {
                                tunnel: w438 -> [w441 w445]
                                tunnel: [w441 w447] -> w437
                                tunnel: w436 -> [_ w448]
                                tunnel: w435 -> [_ w446]
                                tunnel: w434 -> [_ w443]
                                tunnel: w433 -> [_ w444]
                                tunnel: w432 -> [_ w442]
                                frame False {
                                }
                                frame True {
                                n160 = case shown="Default" w442 {
                                tunnel: w448 -> [_ w459]
                                tunnel: [w449 w456] -> w447
                                tunnel: w446 -> [_ w455]
                                tunnel: w445 -> [w449 w453]
                                tunnel: w444 -> [_ w451]
                                tunnel: w443 -> [_ w450]
                                frame -1..1 {
                                }
                                frame Default {
                                n161 = Unbundle By Name(w459) -> ("time"=w457:dbl[], "TagsData"=w458:T3)
                                n162 = call "BIN_make_new_file.vi"("error in"=w453, "TAGs"=w450, "FileName"=w455) -> ("error out"=w452:errorcluster, "refnum out"=w454:refnum<file>)  [unwired: 7 in]
                                n163 = Bundle By Name(cluster=T5 {"TableName"="", "Data2save"={"TAGs"=[], "time"=[], "TagsData"=[]}} ("Data in"), "TableName"=w451, "Data2save.TAGs"=w450, "Data2save.time"=w457, "Data2save.TagsData"=w458) -> (w460:T5)
                                n164 = call "BIN-write.vi"("error in"=w452, "Data in"=w460, "refnum in"=w454) -> ("error out"=w456:errorcluster)  [unwired: 6 in, 2 out]
                                }
                                }
                                }
                                }
                              }
                            }
                          }
                        }
                      }
                      frame Default {
                      }
                    }
                  }
                }
              }
            }
          }
        }
      }
    }
  }
